vi "CANOpen Change PDO Channel.vi"(8 "error in (no error)":errorcluster, 10 "PDO Channel":u8 max=127 step=1, 11 "Node Ptr":u64 format="%.0x") -> (0 "error out":errorcluster, 3 "Passed?":bool)   [LabVIEW 2013]
uses:
  <vilib>/NI Veristand/Custom Device API/Custom Device API.lvlib
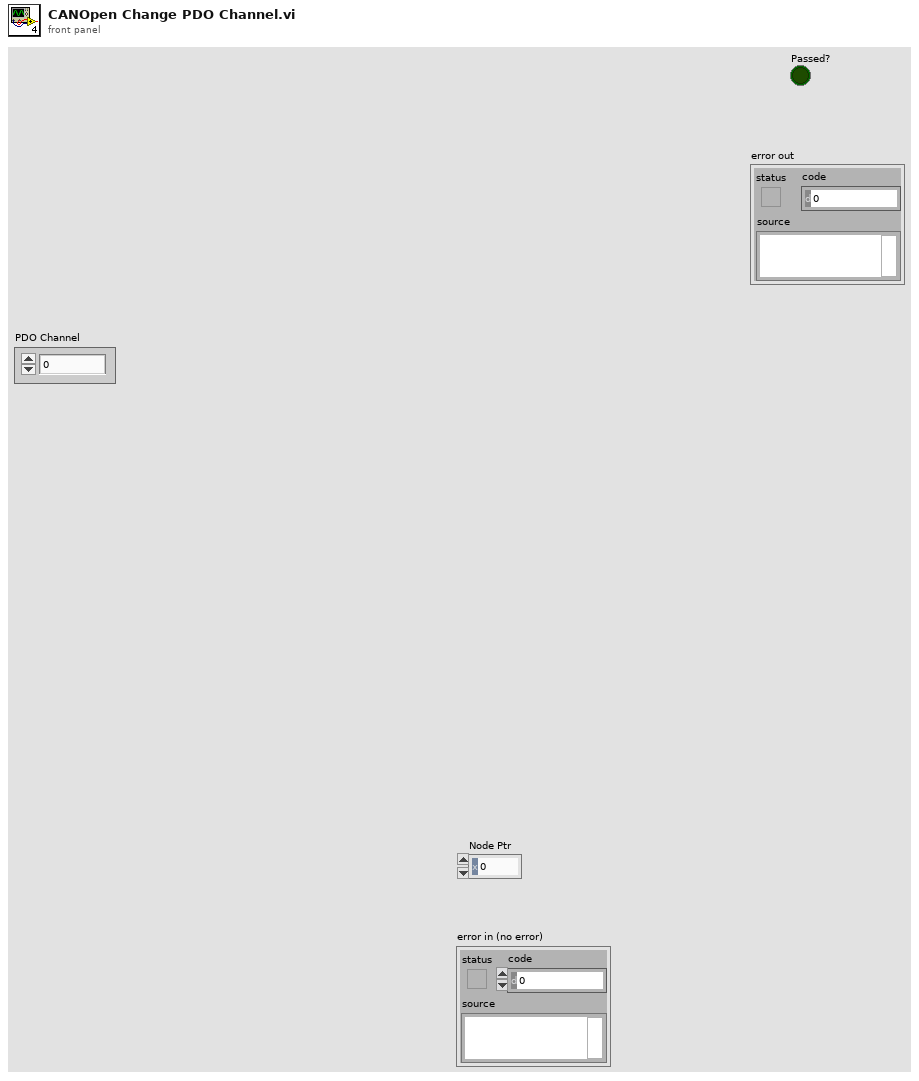
[diagram p1: front panel]
types:
  T1 = typedef "Custom Device API.lvlib/Custom Device Item Ref.ctl" = u64
  T2 = typedef "Custom Device API.lvlib/Custom Device Item Info.ctl" = cluster{"Name":string, "Is Channel":bool, "GUID":string, "Is Waveform":bool}
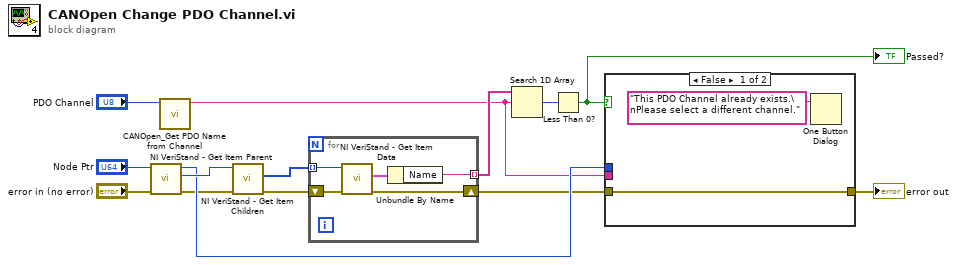
[diagram p0: block diagram]
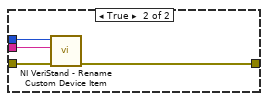
[diagram p2: hidden frame]
diagram:
  n1 = call <vilib>:"NI VeriStand - Get Item Parent.vi"("error in (no error)"="error in (no error)", "Item Ref in"="Node Ptr") -> ("error out"=w4:errorcluster, "Parent Ref"=w8:T1, "Item Ref out"=w6:T1)  [unwired: 6 in, 1 out]
  n2 = call "CANOpen_Get PDO Name from Channel.vi"("PDO Channel"="PDO Channel") -> ("PDO Channel Name"=w2:string)  [unwired: 10 in]
  n3 = call <vilib>:"NI VeriStand - Get Item Children.vi"("error in (no error)"=w4, "Item Ref in"=w8) -> ("error out"=w14:errorcluster, "Child Refs"=w13:T1[])  [unwired: 6 in, 2 out]
  n4 = for {
    tunnel: w13 -> [w18] mode=indexing
    tunnel: [w15] -> w9 mode=indexing
    shift-right: [w16] -> w1
    shift-left: w14 -> [w17]
    n5 = call <vilib>:"NI VeriStand - Get Item Data.vi"("error in (no error)"=w17, "Item Ref in"=w18) -> ("error out"=w16:errorcluster, "Item Info"=w19:T2)  [unwired: 6 in, 2 out]
    n6 = Unbundle By Name(w19) -> ("Name"=w15:string)
  }
  n7 = Search 1D Array(1D array=w9, element=w2) -> (index of element=w10:i32)  [unwired: 1 in]
  n8 = Less Than 0?(x=w10) -> (x < 0?=w11:bool)
  "Passed?" <- w11
  n9 = case shown="False" w11 {
    tunnel: [w20 w24] -> w7
    tunnel: w1 -> [w20 w25]
    tunnel: w2 -> [_ w23]
    tunnel: w6 -> [_ w22]
    frame False {
      n10 = One Button Dialog(message="This PDO Channel already exists.\nPlease select a different channel.") -> ()  [unwired: 1 in, 1 out]
    }
    frame True {
      n11 = call <vilib>:"NI VeriStand - Rename Custom Device Item.vi"("error in (no error)"=w25, "New Name"=w23, "Item Ref in"=w22) -> ("error out"=w24:errorcluster)  [unwired: 1 in, 7 out]
    }
  }
  "error out" <- w7
